vi "timesensorvariable.vi"(9 "Elapsed time in current state":dbl format="%.2f", 10 "S P & V definitions":T3[](array[typedef]) {"value" format="%#_6p"; "variable"."Data average interval" min=0.0 format="%^#_3g"}, 11 "condition":T1 {"Data average interval" min=0.0 format="%^#_3g"; "sensors and variables" items=["Elapsed time in current state"]}) -> (3 "exit":bool)   [LabVIEW 2015]
uses:
  variable setpoint.ctl
  data ave interval.ctl
  type specifier for control code.ctl
  condition.ctl
  greater or less.ctl
  DAQ configuration/Sensor buffer command.ctl
  calibration/Shared Data/share data command.ctl
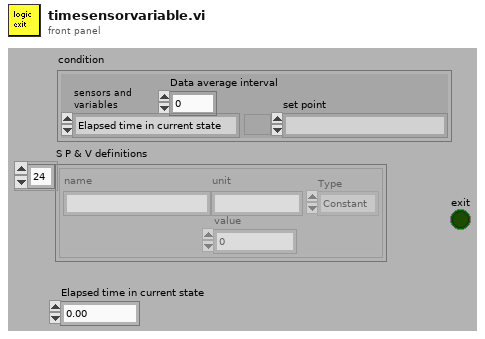
[diagram p1: front panel]
types:
  T1 = typedef "condition.ctl" = cluster{"> or <":T2, "set point":i32, "sensors and variables":i32, "Data average interval":dbl}
  T2 = typedef "greater or less.ctl" = bool
  T3 = typedef "variable setpoint.ctl" = cluster{"name":string, "unit":string, "value":dbl, "Type":enum16{"Constant", "Variable"}, "variable":cluster{"selected sensors":i32[], "selected set points":i32[], "VI":path, "Data average interval":T4, "code ref":T5}}
  T4 = typedef "data ave interval.ctl" = dbl
  T5 = typedef "type specifier for control code.ctl" = refnum<vi>
  T6 = typedef "share data command.ctl" = enum16{"Initialize from ini", "Update ini", "Write data", "Read data", "List my data", "List shared data", "Close"}
  T7 = typedef "Sensor buffer command.ctl" = enum16{"read average", "read recent", "read all", "write", "set buffer size", "Read channel config", "Write channel config", "clear"}
  T8 = typedef "Sensor data.ctl" = cluster{" Sensor array":T9[], "Time":dbl}
  T9 = typedef "sensor cluster.ctl" = cluster{"voltage":sgl, "scaled":sgl, "units":string, "Out of Range":bool}
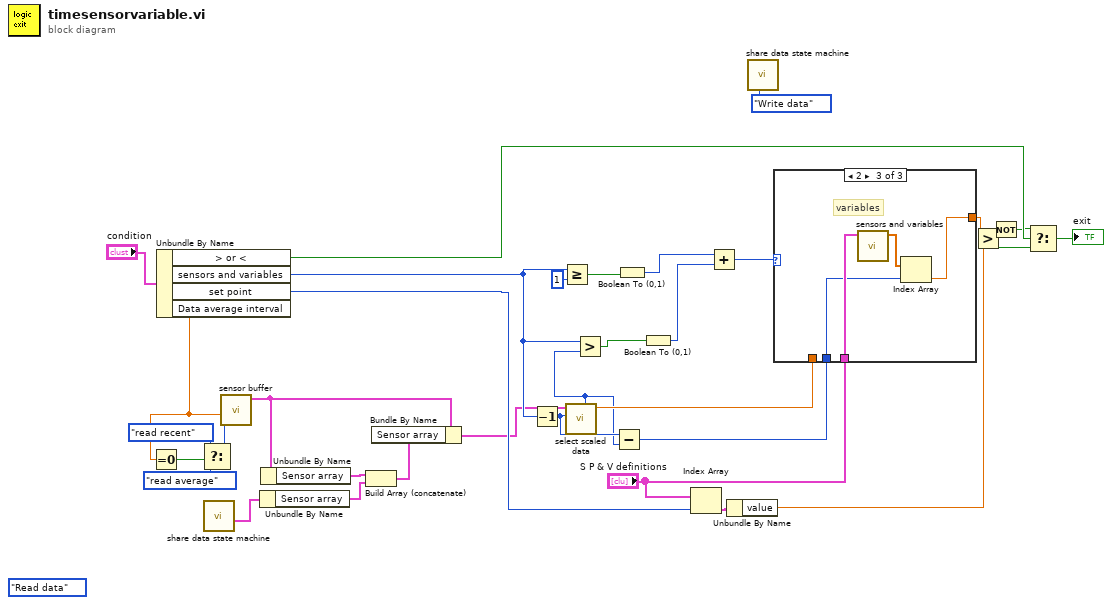
[diagram p0: block diagram]
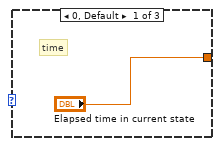
[diagram p2: hidden frame]
diagram:
  (unwired) share_data_command."Read data" ("Share data command")
  n1 = Unbundle By Name("condition") -> ("> or <"=w19:T2, "sensors and variables"=w25:i32, "set point"=w22:i32, "Data average interval"=w27:dbl)
  n2 = Equal To 0?(x=w27) -> (x = 0?=w32:bool)
  n3 = Select(t=Sensor_buffer_command."read recent" ("command"), s=w32, f=Sensor_buffer_command."read average" ("command")) -> (s? t:f=w31:T7)
  n4 = call "share data state machine.vi"() -> ("Data from shared sources"=w6:T8)  [unwired: 5 in, 6 out]
  n5 = call "sensor buffer.vi"("command"=w31, "smooth interval (s)"=w27) -> ("Calibrated data"=w3:T8)  [unwired: 5 in, 4 out]
  n6 = Unbundle By Name(w6) -> ("Sensor array"=w4:T9[])
  n7 = Unbundle By Name(w3) -> ("Sensor array"=w5:T9[])
  n8 = Build Array (concatenate)(w5, w4) -> (w2:T9[])
  n9 = Bundle By Name(cluster=w3, "Sensor array"=w2) -> (w1:T8)
  n10 = Decrement(x=w25) -> (x-1=w12:i32)
  n11 = Greater Or Equal?(x=w25, y=1) -> (x >= y?=w33:bool)
  n12 = call "select scaled data.vi"("Sensor index"=w12, "Sensor Data"=w1) -> ("scaled"=w26:sgl, "number of sensors"=w11:i32)  [unwired: 4 in, 4 out]
  n13 = Greater?(x=w25, y=w11) -> (0:w8:bool)
  n14 = Subtract(x=w12, y=w11) -> (x-y=w10:i32)
  n15 = Boolean To (0,1)(Boolean=w33) -> (0, 1=w16:i16)
  n16 = Boolean To (0,1)(Boolean=w8) -> (0, 1=w15:i16)
  n17 = Index Array(array="S P & V definitions", index=w22) -> (element=w24:T3)
  n18 = Add(x=w16, y=w15) -> (x+y=w9:i16)
  n19 = Unbundle By Name(w24) -> ("value"=w21:dbl)
  n20 = call "share data state machine.vi"("Share data command"=share_data_command."Write data") -> ()  [unwired: 4 in, 7 out]
  n21 = case shown="2" w9 {
    tunnel: w26 -> [_ w35 _]
    tunnel: ["Elapsed time in current state" w35 w38] -> w20
    tunnel: "S P & V definitions" -> [_ _ w37]
    tunnel: w10 -> [_ _ w36]
    frame 0, Default {
      # "time"
    }
    frame 1 {
      # "sensors"
    }
    frame 2 {
      # "variables"
      n22 = call "sensors and variables.vi"("S P & V definitions"=w37) -> ("Variable values"=w39:dbl[])  [unwired: 6 in, 4 out]
      n23 = Index Array(array=w39, index=w36) -> (element=w38:dbl)
    }
  }
  n24 = Greater?(x=w20, y=w21) -> (0:w14:bool)
  n25 = Not(x=w14) -> (.not. x?=w13:bool)
  n26 = Select(t=w13, s=w19, f=w14) -> (s? t:f=→"exit":bool)
